vi "TDMSToDetectedPeaks.vi"(11 "Array":dbl[][](array[numeric])) -> (3 "Detected peaks":T1[](array[typedef]))   [LabVIEW 2021]
uses:
  Typedefs/Detected peaks.ctl
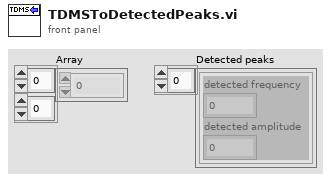
[diagram p1: front panel]
types:
  T1 = typedef "Detected peaks.ctl" = cluster{"detected frequency":dbl, "detected amplitude":dbl}
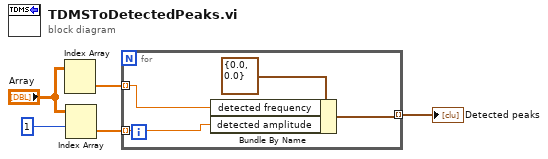
[diagram p0: block diagram]
diagram:
  n1 = Index Array(array="Array") -> (element=w3:dbl[])  [unwired: 2 in]
  n2 = Index Array(array="Array", index (row)=1) -> (element=w2:dbl[])  [unwired: 1 in]
  n3 = for {
    tunnel: w3 -> [w8] mode=indexing
    tunnel: w2 -> [w7] mode=indexing
    tunnel: [w6] -> w1 mode=indexing
    n4 = Bundle By Name(cluster=T1 {"detected frequency"=0.0, "detected amplitude"=0.0}, "detected frequency"=w8, "detected amplitude"=w7) -> (w6:T1)
  }
  "Detected peaks" <- w1
